vi "LoadFromFile.vi"(8 "error in (no error)":errorcluster, 10 "path":path, 11 "CoeFile in":refnum<class "CoeFile.lvclass">) -> (0 "error out":errorcluster, 3 "CoeFile out":refnum<class "CoeFile.lvclass">)   [LabVIEW 2013, in "CoeFile.lvclass"]
uses:
  CoeFile.lvclass
  CoeFile.lvclass/CoeFile.ctl
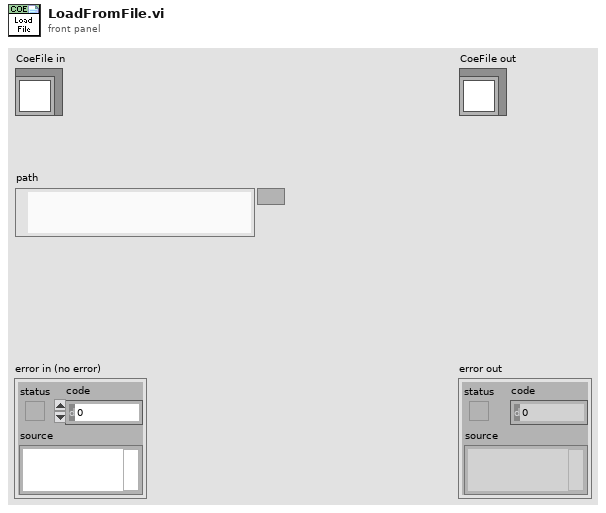
[diagram p1: front panel]
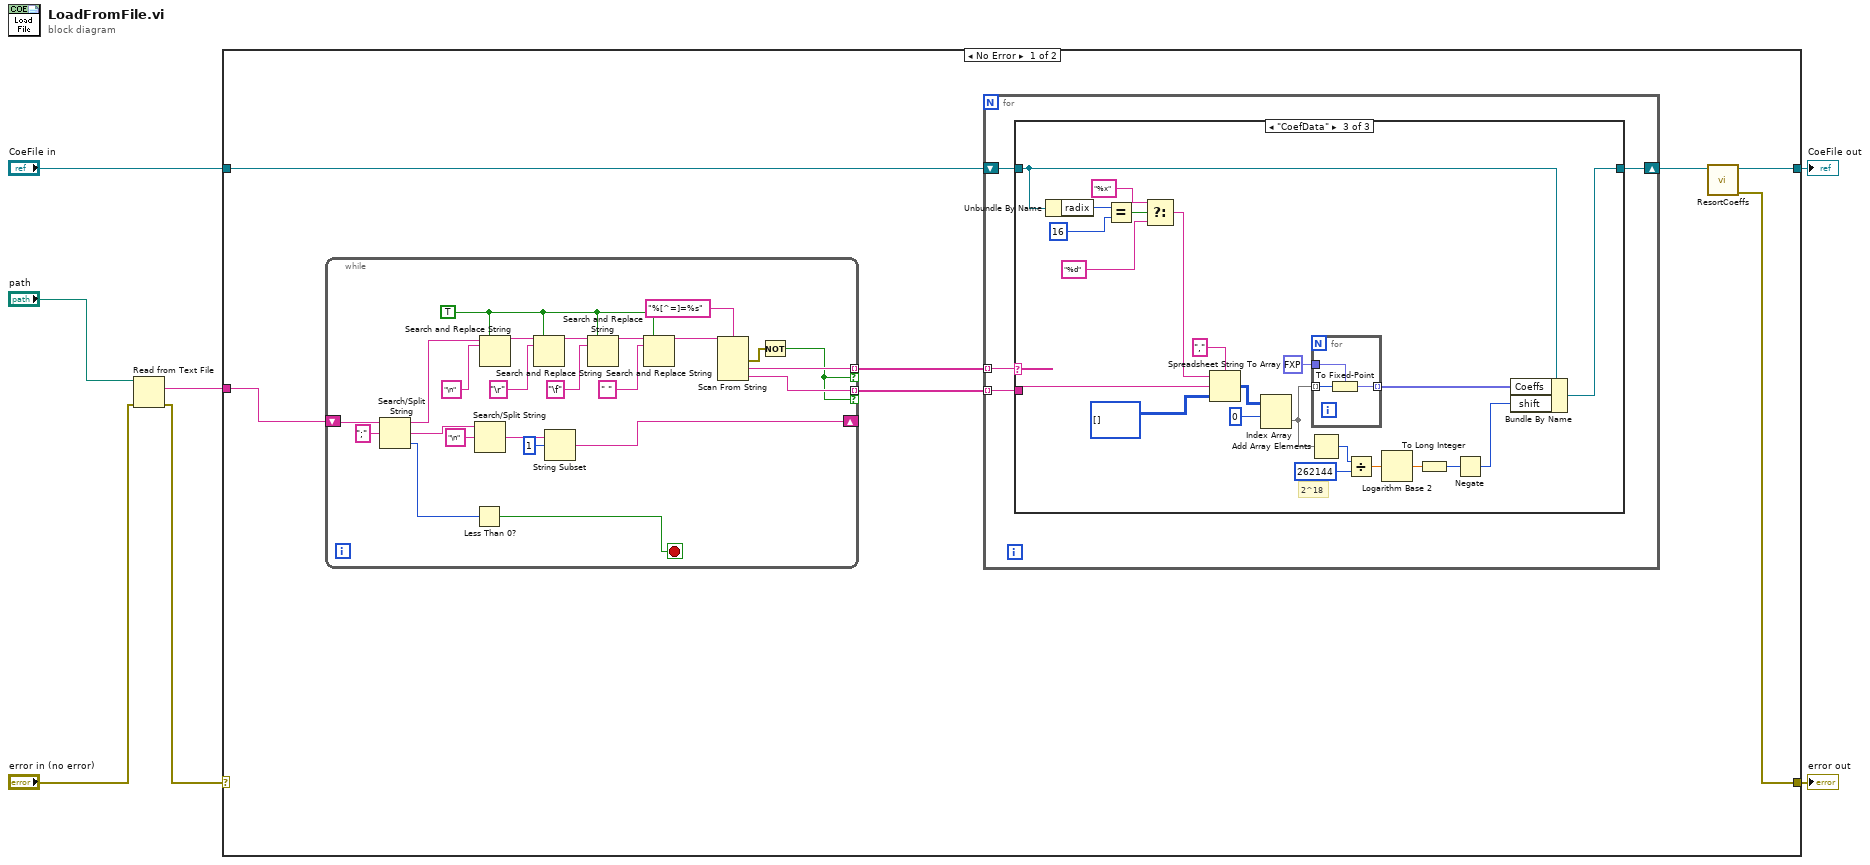
[diagram p0: block diagram]
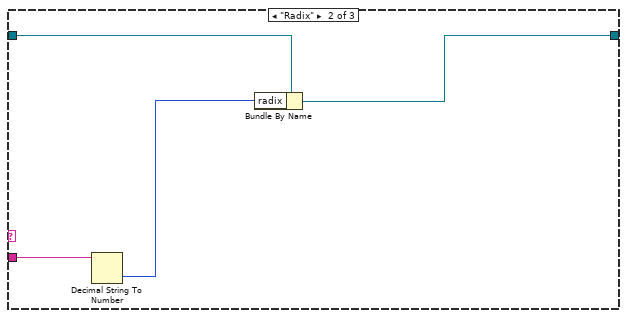
[diagram p3: hidden frame]
diagram:
  n1 = Read from Text File(file (use dialog)="path", error in="error in (no error)") -> (text=w2:string, error out=w3:errorcluster)  [unwired: 2 in, 2 out]
  n2 = case shown="No Error" w3 {
    selector: w3 -> [_ w74]
    tunnel: [w9 w74] -> w7
    tunnel: [w10 w73] -> w5
    tunnel: "CoeFile in" -> [w11 w73]
    tunnel: w2 -> [w12 _]
    frame No Error {
      n3 = while {
        shift-right: [w66] -> _
        shift-left: w12 -> [w72]
        tunnel: [w53] -> w14 mode=indexing if=w50
        tunnel: [w51] -> w13 mode=indexing if=w50
        stop <- w64 stop-if-true
        w61 = TRUE ("replace all? (F)")
        n4 = Search/Split String(string=w72, search string/char (-)=";") -> (substring before match=w63:string, match + rest of string=w70:string, offset of match=w65:i32)  [unwired: 1 in]
        n5 = Less Than 0?(x=w65) -> (x < 0?=w64:bool)
        n6 = Search/Split String(string=w70, search string/char (-)="\n") -> (match + rest of string=w68:string)  [unwired: 1 in, 2 out]
        n7 = Search and Replace String(replace all?=w61, input string=w63, search string="\n" ("search string/char (-)")) -> (result string=w55:string)  [unwired: 5 in, 3 out]
        n8 = Search and Replace String(replace all?=w61, input string=w55, search string="\r" ("search string/char (-)")) -> (result string=w56:string)  [unwired: 5 in, 3 out]
        n9 = String Subset(string=w68, offset (0)=1) -> (substring=w66:string)  [unwired: 1 in]
        n10 = Search and Replace String(replace all?=w61, input string=w56, search string="\f" ("search string/char (-)")) -> (result string=w57:string)  [unwired: 5 in, 3 out]
        n11 = Search and Replace String(replace all?=w61, input string=w57, search string=" " ("search string/char (-)")) -> (result string=w49:string)  [unwired: 5 in, 3 out]
        n12 = Scan From String(format string="%[^=]=%s", input string=w49) -> (error out=w52:errorcluster, output 1=w53:string, output 2=w51:string)  [unwired: 4 in, 2 out]
        n13 = Not(x=w52) -> (.not. x?=w50:bool)
      }
      n14 = for {
        tunnel: w14 -> [w18] mode=indexing
        tunnel: w13 -> [w17] mode=indexing
        shift-right: [w15] -> w8
        shift-left: w11 -> [w16]
        n15 = case shown="\"CoefData\"" w18 {
          tunnel: w17 -> [_ w23 w45]
          tunnel: w16 -> [w19 w22 w25]
          tunnel: [w19 w20 w24] -> w15
          frame "False", Default {
          }
          frame "Radix" {
            n16 = Decimal String To Number(string=w23) -> (number=w21:i32)  [unwired: 2 in, 1 out]
            n17 = Bundle By Name(cluster=w22, "radix"=w21) -> (w20:refnum<class "CoeFile.lvclass">)
          }
          frame "CoefData" {
            # "2^18"
            n18 = Unbundle By Name(w25) -> ("radix"=w28:i32)
            n19 = Equal?(x=w28, y=16 ("x")) -> (x = y?=w39:bool)
            n20 = Select(t="%x" ("delimiter (Tab)"), s=w39, f="%d" ("delimiter (Tab)")) -> (s? t:f=w38:string)
            n21 = Spreadsheet String To Array(delimiter (Tab)=",", format string=w38, spreadsheet string=w45, array type (2D Dbl)=i32[][] []) -> (array=w37:i32[][])
            n22 = Index Array(array=w37, index (row)=0 ("disabled index (col)")) -> (element=w29:i32[])  [unwired: 1 in]
            n23 = Add Array Elements(numeric array=w29) -> (sum=w31:i32)
            n24 = for {
              tunnel: w29 -> [w48] mode=indexing
              tunnel: [w47] -> w26 mode=indexing
              tunnel: fxp<+/-,18,18> 0.0 ("fixed-point type") -> [w46]
              n25 = To Fixed-Point(fixed-point type=w46, number=w48) -> (fixed-point=w47:fxp<+/-,18,18>)
            }
            n26 = Divide(x=w31, y=262144 ("sum 0.5")) -> (x/y=w33:dbl)
            n27 = Logarithm Base 2(1:w33) -> (0:w34:dbl)
            n28 = To Long Integer(number=w34) -> (32bit integer=w32:i32)
            n29 = Negate(x=w32) -> (-x=w27:i32)
            n30 = Bundle By Name(cluster=w25, "Coeffs"=w26, "shift"=w27) -> (w24:refnum<class "CoeFile.lvclass">)
          }
        }
      }
      n31 = call "ResortCoeffs.vi"("CoeFile in"=w8) -> ("error out"=w9:errorcluster, "CoeFile out"=w10:refnum<class "CoeFile.lvclass">)  [unwired: 9 in]
    }
    frame Error {
    }
  }
  "error out" <- w7
  "CoeFile out" <- w5
